vi "niDTS BT Dut Rx Abort.vi"(0 "BT Dut Handle in":T1, 11 "error in (no error)":errorcluster) -> (4 "BT Dut Handle out":T1, 15 "error out":errorcluster)   [LabVIEW 2015, in "niDTS BT.lvlib"]
uses:
  niDTS BT.lvlib
  Framework/Dut/Includes/niDTS Dut INC Handle.ctl
  Framework/Dut/Objects/BASE_class/niDTS Dut.lvclass
  Includes/niDTS BT Dut INC Handle.ctl
  Objects/BASE_class/niDTS BT Dut.lvclass
  Framework/niDTS Framework.lvlib
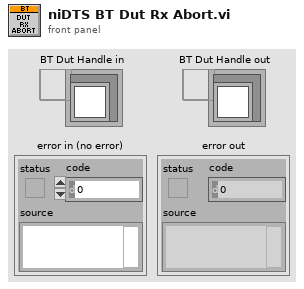
[diagram p1: front panel]
types:
  T1 = typedef "niDTS Framework.lvlib/niDTS Dut INC Handle.ctl" = refnum<data-value>
  T2 = typedef "niDTS BT.lvlib/niDTS BT Dut INC Handle.ctl" = refnum<data-value>
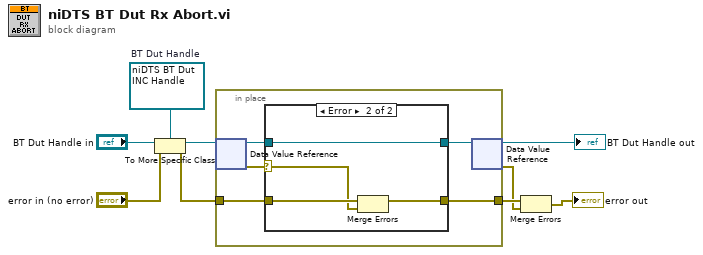
[diagram p0: block diagram]
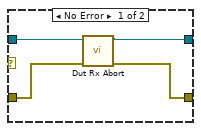
[diagram p2: hidden frame]
diagram:
  w4 = T2 refnum  # BT Dut Handle
  n1 = To More Specific Class(target class=w4, reference="BT Dut Handle in", error in="error in (no error)") -> (specific class reference=w7:T2, error out=w5:errorcluster)
  n2 = in-place {
    in-place-border: w5 -> [w11]
    in-place-border: [w10] -> w3
    n3 = in-place-dvr #1(w7) -> (w13:refnum<class "niDTS BT Dut.lvclass">, w14:errorcluster)
    n4 = case shown="Error" w14 {
      selector: w14 -> [_ w20]
      tunnel: w13 -> [w18 w22]
      tunnel: [w17 w22] -> w12
      tunnel: w11 -> [w16 w21]
      tunnel: [w15 w19] -> w10
      frame No Error {
        n5 = call-dynamic "Dut Rx Abort.vi"("niDTS DUT in"=w18, "error in (no error)"=w16) -> ("niDTS DUT out"=w17:refnum<class "niDTS BT Dut.lvclass">, "error out"=w15:errorcluster)  [unwired: 12 in]
      }
      frame Error {
        n6 = Merge Errors(w21, w20) -> (w19:errorcluster)
      }
    }
    n7 = in-place-dvr #1(w12) -> (→"BT Dut Handle out":T2, w1:errorcluster)
  }
  n8 = Merge Errors(w3, w1) -> (→"error out":errorcluster)
